vi "关键参数组合 (子VI).vi"(10 "因子编码":string, 11 "DO":string[](array[string])) -> (3 "字符串":string)   [LabVIEW 2016, in "数据传输系统.lvlib"]
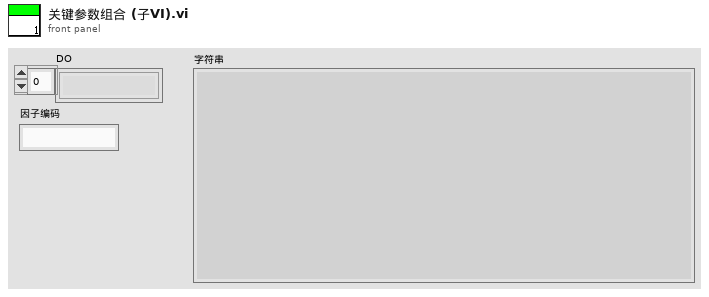
[diagram p1: front panel]
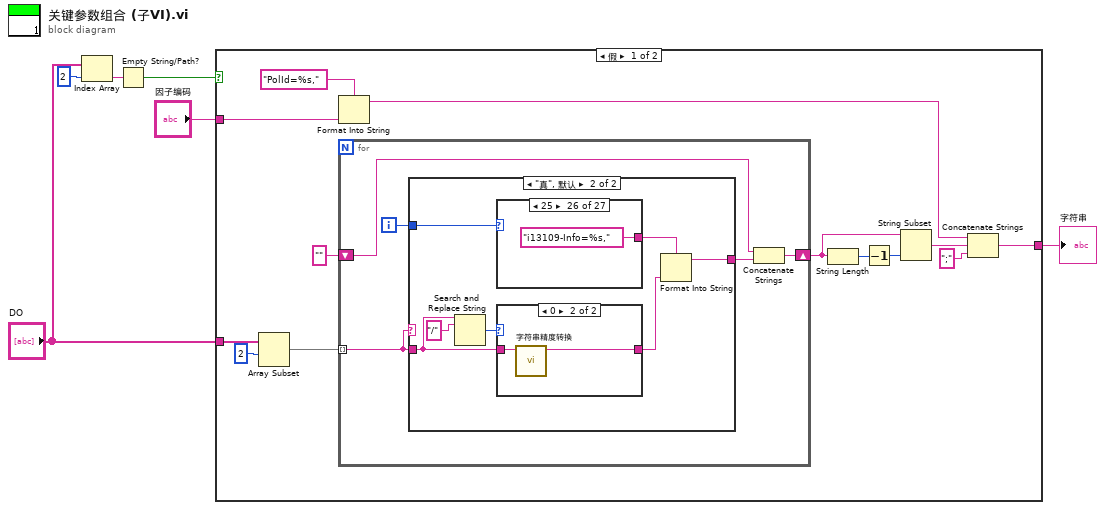
[diagram p0: block diagram]
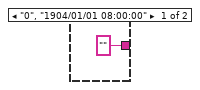
[diagram p2: hidden frame]
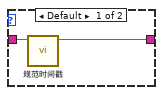
[diagram p3: hidden frame]
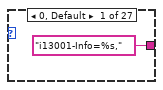
[diagram p4: hidden frame]
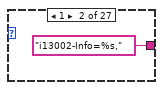
[diagram p5: hidden frame]
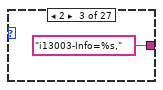
[diagram p6: hidden frame]
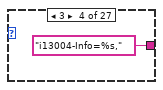
[diagram p7: hidden frame]
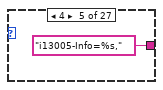
[diagram p8: hidden frame]
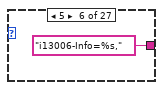
[diagram p9: hidden frame]
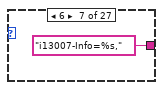
[diagram p10: hidden frame]
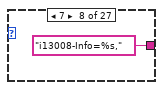
[diagram p11: hidden frame]
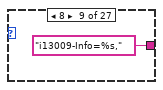
[diagram p12: hidden frame]
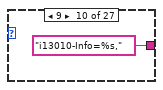
[diagram p13: hidden frame]
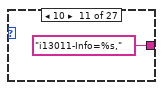
[diagram p14: hidden frame]
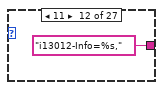
[diagram p15: hidden frame]
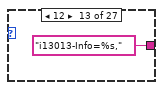
[diagram p16: hidden frame]
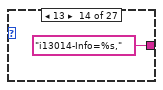
[diagram p17: hidden frame]
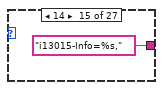
[diagram p18: hidden frame]
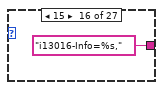
[diagram p19: hidden frame]
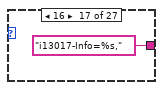
[diagram p20: hidden frame]
diagram:
  n1 = Index Array(array="DO", index=2 ("索引")) -> (element=w5:string)
  n2 = Empty String/Path?(string/path=w5) -> (empty?=w4:bool)
  n3 = case shown="假" w4 {
    tunnel: [w13 ""] -> w3
    tunnel: "DO" -> [w12 _]
    tunnel: "因子编码" -> [w8 _]
    frame False {
      n4 = Array Subset(array=w12, index=2 ("索引")) -> (w10:string[])  [unwired: 1 in]
      n5 = Format Into String(format string="PolId=%s,", w8) -> (resulting string=w7:string)  [unwired: 2 in, 1 out]
      n6 = for {
        shift-right: [w21] -> w17
        shift-left: "" -> [w23]
        tunnel: w10 -> [w20] mode=indexing
        i -> [w24]
        n7 = case shown="\"真\", 默认" w20 {
          tunnel: w24 -> [_ w32]
          tunnel: ["" w30] -> w22
          tunnel: w20 -> [_ w27]
          frame "0", "1904/01/01 08:00:00" {
          }
          frame "真", Default {
            n8 = Search and Replace String(input string=w27, search string="/" ("搜索字符串")) -> (number of replacements=w29:i32)  [unwired: 6 in, 3 out]
            n9 = case shown="25" w32 {
              tunnel: ["i13001-Info=%s," "i13002-Info=%s," "i13003-Info=%s," "i13004-Info=%s," "i13005-Info=%s," "i13006-Info=%s," "i13007-Info=%s," "i13008-Info=%s," "i13009-Info=%s," "i13010-Info=%s," "i13011-Info=%s," "i13012-Info=%s," "i13013-Info=%s," "i13014-Info=%s," "i13015-Info=%s," "i13016-Info=%s," "i13017-Info=%s," "i13101-Info=%s," "i13102-Info=%s," "i13103-Info=%s," "i13104-Info=%s," "i13105-Info=%s," "i13106-Info=%s," "i13107-Info=%s," "i13108-Info=%s," "i13109-Info=%s," "i13110-Info=%s,"] -> w31
              frame 0, Default {
              }
              frame 1 {
              }
              frame 2 {
              }
              frame 3 {
              }
              frame 4 {
              }
              frame 5 {
              }
              frame 6 {
              }
              frame 7 {
              }
              frame 8 {
              }
              frame 9 {
              }
              frame 10 {
              }
              frame 11 {
              }
              frame 12 {
              }
              frame 13 {
              }
              frame 14 {
              }
              frame 15 {
              }
              frame 16 {
              }
              frame 17 {
              }
              frame 18 {
              }
              frame 19 {
              }
              frame 20 {
              }
              frame 21 {
              }
              frame 22 {
              }
              frame 23 {
              }
              frame 24 {
              }
              frame 25 {
              }
              frame 26 {
              }
            }
            n10 = case shown="0" w29 {
              tunnel: w27 -> [w34 w36]
              tunnel: [w33 w35] -> w26
              frame Default {
                n11 = call "规范时间戳.vi"("字符串"=w34) -> ("result string"=w33:string)  [unwired: 10 in]
              }
              frame 0 {
                n12 = call "字符串精度转换.vi"("输入字符串"=w36) -> ("输出字符串"=w35:string)  [unwired: 9 in, 1 out]
              }
            }
            n13 = Format Into String(format string=w31, w26) -> (resulting string=w30:string)  [unwired: 2 in, 1 out]
          }
        }
        n14 = Concatenate Strings(w23, w22) -> (w21:string)
      }
      n15 = String Length(string=w17) -> (length=w16:i32)
      n16 = Decrement(x=w16) -> (x-1=w15:i32)
      n17 = String Subset(string=w17, length (rest)=w15) -> (substring=w14:string)  [unwired: 1 in]
      n18 = Concatenate Strings(w7, w14, ";") -> (w13:string)
    }
    frame True {
    }
  }
  "字符串" <- w3
